vi "Read Section - Timestamp.vi"(4 "Default":timestamp, 6 "Create file if not found? (T)":bool=TRUE, 8 "error in (no error)":errorcluster, 9 "key":string, 10 "section":string, 11 "Path":path) -> (0 "error out":errorcluster, 3 "Value":timestamp)   [LabVIEW 2019, in "TSC File IO.lvlib"]
doc: "This VI will read a section/cluster configuration file and return type timestamp.\n\nInputs:\n-Path [path] - a path to the file\n-section [string] - the section string in the configuration file\n-key [string] - the key to be read in the configuration file\n-error in\n\nOutputs:\n-value [timestamp] - the output data read\n-error out\n_________________________________________________________________________\n<b>Code Developed By:</b>\nDaniel Coons\nTechnology Service Corporation\n1983 S Liberty Drive\nBloomington, IN 47403\nPhone: 812 558-7100\ndaniel.coons@tsc.com\nwww.tsc.com\n\n<b>Date Created:</b> 05 SEP 2014\n<b>Date Updated:</b> 13 APR 2020"
uses:
  TSC File IO.lvlib
  <vilib>/Utility/config.llb/NI_LVConfig.lvlib
  <vilib>/Utility/config.llb/Read Key (String).vi
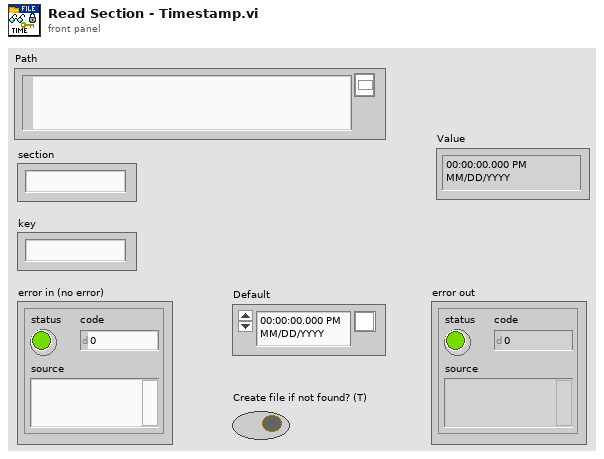
[diagram p1: front panel]
types:
  T1 = typedef "NI_LVConfig.lvlib/Config Data RefNum.ctl" = refnum<k1>
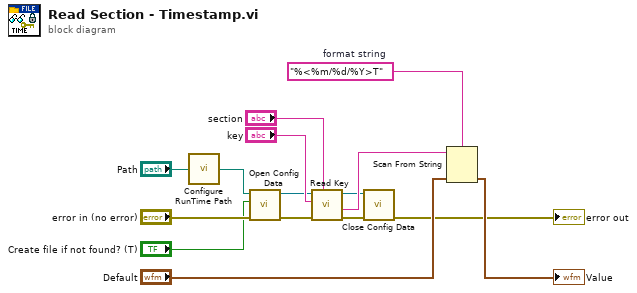
[diagram p0: block diagram]
diagram:
  w6 = "%<%m/%d/%Y>T"  # format string
  n1 = call "Configure RunTime Path.vi"("Input Path"="Path") -> ("Updated Path"=w5:path)
  n2 = call <vilib>:"Open Config Data.vi"("error in (no error)"="error in (no error)", "create file if necessary (T)"="Create file if not found? (T)", "configuration file path"=w5) -> ("error out"=w8:errorcluster, "refnum"=w9:T1)  [unwired: 6 in, 1 out]
  n3 = call-poly <vilib>:"Read Key.vi"("section"="section", "error in (no error)"=w8, "key"="key", "refnum"=w9) -> ("error out"=w10:errorcluster, "value"=w12:string, "refnum out"=w11:T1)  [unwired: 4 in, 1 out]
  n4 = call <vilib>:"Close Config Data.vi"("error in (no error)"=w10, "refnum"=w11) -> ("error out"=→"error out":errorcluster)  [unwired: 8 in, 1 out]
  n5 = Scan From String(format string=w6, input string=w12, default 1="Default") -> (output 1=→"Value":timestamp)  [unwired: 2 in, 3 out]
